vi "operaciones.vi"() -> ()   [LabVIEW 2017]
panel:
  out "A / B":dbl format="%#.1f"
  out "A * B":dbl
  out "A - B":dbl
  out "A + B":dbl
  in  "B":dbl
  in  "A":dbl
  out "Esta es la fecha de hoy":timestamp
  # "Dato B"
  # "Dato A"
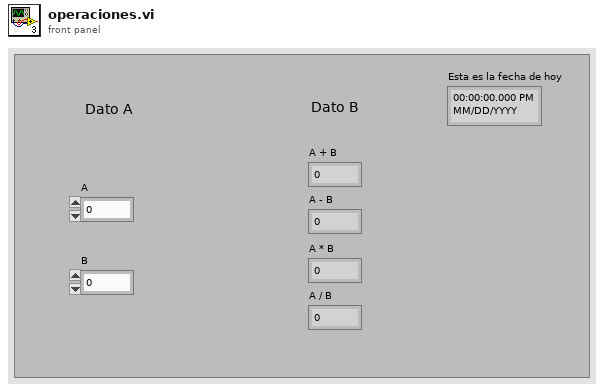
[diagram p1: front panel]
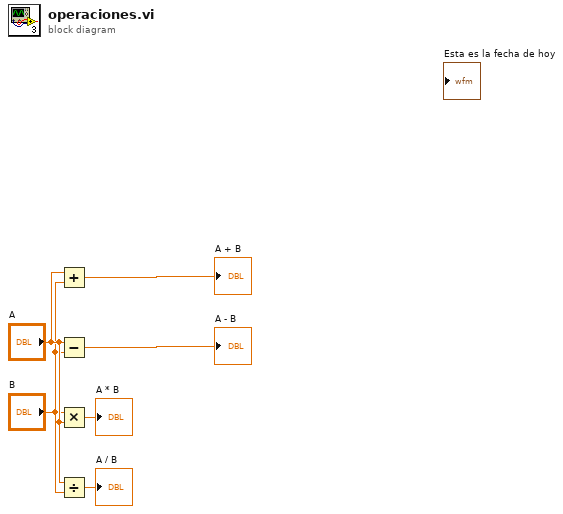
[diagram p0: block diagram]
diagram:
  n1 = Add(x="A", y="B") -> (x+y=→"A + B":dbl)
  n2 = Subtract(x="A", y="B") -> (x-y=→"A - B":dbl)
  n3 = Multiply(x="B", y="A") -> (x*y=→"A * B":dbl)
  n4 = Divide(x="A", y="B") -> (x/y=→"A / B":dbl)
